vi "Helper SubVI - Spectral Subtraction.vi"(4 "attenuation factor":dbl, 5 "Enhance?":bool, 6 "noise level":dbl, 7 "reset":bool, 11 "Gabor coefficients in":cdb[][](array[numeric])) -> (3 "Gabor coefficients out":cdb[][](array[numeric]))   [LabVIEW 2023]
doc: "Generate the enhanced Gabor coefficents according to the noise level and attenuation factor."
panel:
  in  "buffer size":i32=5
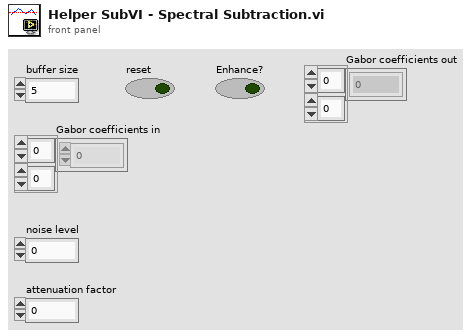
[diagram p1: front panel]
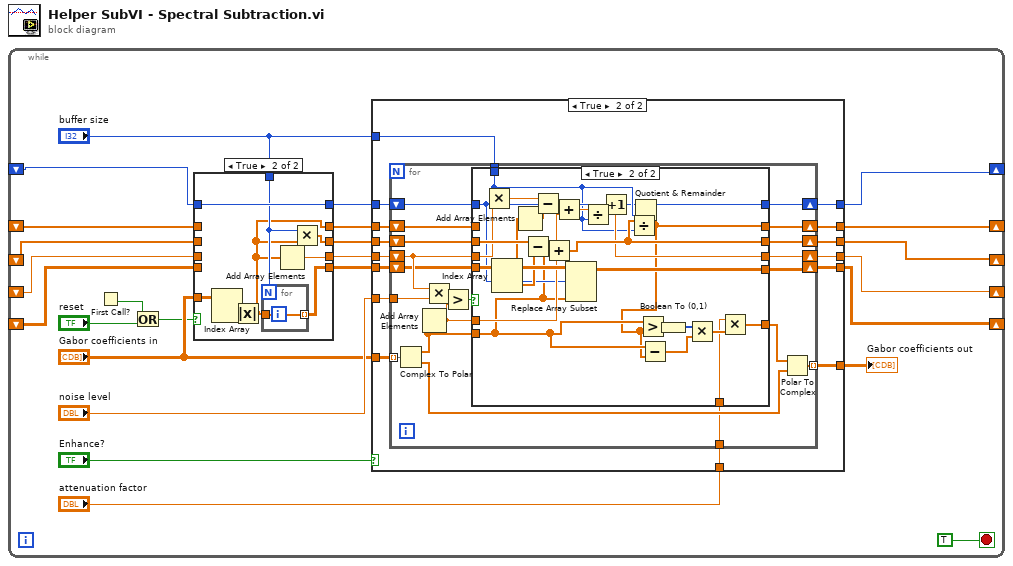
[diagram p0: block diagram]
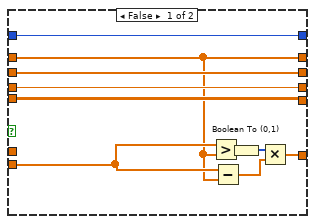
[diagram p3: hidden frame]
diagram:
  n1 = while {
    shift-right: [w12] -> _
    shift-left: _ -> [w6]
    shift-right: [w11] -> _
    shift-left: _ -> [w5]
    shift-right: [w10] -> _
    shift-left: _ -> [w4]
    shift-right: [w9] -> _
    shift-left: _ -> [w3]
    shift-right: [w8] -> _
    shift-left: _ -> [w7]
    stop <- TRUE stop-if-true
    n2 = First Call?() -> (First Call?: T/F=w1:bool)
    n3 = Or(x=w1, y="reset") -> (x .or. y?=w2:bool)
    n4 = case shown="True" w2 {
      tunnel: "Gabor coefficients in" -> [_ w115]
      tunnel: w3 -> [w107 _]
      tunnel: [w107 w114] -> w15
      tunnel: w5 -> [w106 _]
      tunnel: [w106 w109] -> w14
      tunnel: "buffer size" -> [_ w110]
      tunnel: [w104 w112] -> w16
      tunnel: w7 -> [w105 w111]
      tunnel: [w105 w111] -> w17
      tunnel: w4 -> [w104 _]
      tunnel: w6 -> [w103 _]
      tunnel: [w103 w108] -> w19
      frame False {
      }
      frame True {
        n5 = Index Array(array=w115) -> (element=w113:cdb[])  [unwired: 2 in]
        n6 = Absolute Value(x=w113) -> (abs(x)=w108:dbl[])
        n7 = for {
          N: w110 -> [_]
          tunnel: w108 -> [w116]
          tunnel: [w116] -> w114 mode=indexing
        }
        n8 = Add Array Elements(numeric array=w108) -> (sum=w112:dbl)
        n9 = Multiply(x=w110, y=w108) -> (x*y=w109:dbl[])
      }
    }
    n10 = case shown="True" "Enhance?" {
      tunnel: "Gabor coefficients in" -> [w27 w46]
      tunnel: w14 -> [w30 w45]
      tunnel: w15 -> [w28 w44]
      tunnel: w16 -> [w29 w43]
      tunnel: w17 -> [w26 w42]
      tunnel: "buffer size" -> [_ w41]
      tunnel: [w30 w40] -> w11
      tunnel: [w29 w39] -> w10
      tunnel: [w28 w38] -> w9
      tunnel: w19 -> [w31 w37]
      tunnel: [w31 w36] -> w12
      tunnel: [w27 w35] -> w22
      tunnel: [w26 w34] -> w8
      tunnel: "noise level" -> [_ w33]
      tunnel: "attenuation factor" -> [_ w32]
      frame False {
      }
      frame True {
        n11 = for {
          tunnel: w46 -> [w65] mode=indexing
          shift-right: [w56] -> w38
          shift-left: w44 -> [w62]
          shift-right: [w58] -> w39
          shift-left: w43 -> [w63]
          shift-right: [w57] -> w40
          shift-left: w45 -> [w64]
          shift-right: [w52] -> w34
          shift-left: w42 -> [w61]
          tunnel: w41 -> [w60]
          shift-right: [w50] -> w36
          shift-left: w37 -> [w55]
          tunnel: [w53] -> w35 mode=indexing
          tunnel: w33 -> [w48]
          tunnel: w32 -> [w47]
          n12 = Complex To Polar(r * e^(i*theta)=w65) -> (r=w51:dbl[], theta=w54:dbl[])
          n13 = Add Array Elements(numeric array=w51) -> (sum=w59:dbl)
          n14 = Multiply(x=w63, y=w48) -> (x*y=w67:dbl)
          n15 = Greater?(x=w67, y=w59) -> (0:w66:bool)
          n16 = case shown="True" w66 {
            tunnel: w51 -> [w70 w82]
            tunnel: w64 -> [w69 w100]
            tunnel: w63 -> [w77 w99]
            tunnel: w62 -> [w76 w102]
            tunnel: w61 -> [w75 w89]
            tunnel: w60 -> [_ w88]
            tunnel: w59 -> [_ w94]
            tunnel: [w77 w90] -> w58
            tunnel: [w69 w91] -> w57
            tunnel: [w76 w92] -> w56
            tunnel: w55 -> [w68 _]
            tunnel: [w68 w81] -> w50
            tunnel: [w75 w86] -> w52
            tunnel: [w71 w79] -> w49
            tunnel: w47 -> [_ w78]
            frame False {
              n17 = Greater?(x=w70, y=w68) -> (0:w72:bool[])
              n18 = Subtract(x=w70, y=w68) -> (x-y=w74:dbl[])
              n19 = Boolean To (0,1)(Boolean=w72) -> (0, 1=w73:i16[])
              n20 = Multiply(x=w73, y=w74) -> (x*y=w71:dbl[])
            }
            frame True {
              n21 = Multiply(x=w88, y=w99) -> (x*y=w98:dbl)
              n22 = Index Array(array=w102, index (row)=w89) -> (element=w96:dbl[])  [unwired: 1 in]
              n23 = Add Array Elements(numeric array=w96) -> (sum=w97:dbl)
              n24 = Subtract(x=w100, y=w96) -> (x-y=w101:dbl[])
              n25 = Subtract(x=w98, y=w97) -> (x-y=w95:dbl)
              n26 = Add(x=w101, y=w82) -> (x+y=w91:dbl[])
              n27 = Add(x=w95, y=w94) -> (x+y=w93:dbl)
              n28 = Replace Array Subset(array=w102, new element=w82, index (row)=w89) -> (w92:dbl[][])  [unwired: 1 in]
              n29 = Divide(x=w93, y=w88) -> (x/y=w90:dbl)
              n30 = Increment(x=w89) -> (x+1=w87:i32)
              n31 = Divide(x=w91, y=w88) -> (x/y=w81:dbl[])
              n32 = Quotient & Remainder(x=w87, y=w88) -> (x-y*floor(x/y)=w86:i32)  [unwired: 1 out]
              n33 = Greater?(x=w82, y=w81) -> (0:w83:bool[])
              n34 = Subtract(x=w82, y=w81) -> (x-y=w85:dbl[])
              n35 = Boolean To (0,1)(Boolean=w83) -> (0, 1=w84:i16[])
              n36 = Multiply(x=w84, y=w85) -> (x*y=w80:dbl[])
              n37 = Multiply(x=w78, y=w80) -> (x*y=w79:dbl[])
            }
          }
          n38 = Polar To Complex(1:w54, 2:w49) -> (0:w53:cdb[])
        }
      }
    }
    "Gabor coefficients out" <- w22
  }
